vi "Word_doc.vi"(4 "end":i32, 6 "start":i32, 7 "insertion point":u16(ring)=1 items=["begining of document", "end of document", "bookmark", "Custom"], 8 "error in (no error)":errorcluster, 9 "report file path out":path=path "C:/Users/Joseph/Desktop/New folder/5.docx", 10 "Report in 2":path=path "C:/Users/Joseph/Desktop/RRATP000001 ATP_NAMER_60A_BDLC_60A _Vers 10_160816.doc", 11 "Report in 1":path=path "C:/KineticksTester/N30_00000_200817_1048.docx") -> (0 "error out":errorcluster)   [LabVIEW 2017]
uses:
  <vilib>/Utility/NIReport.llb/NI_report.lvclass
  <vilib>/Utility/NIReport.llb/Word/NI_Word.lvclass
  <vilib>/addons/_office/NI_ReportGenerationToolkit.lvlib
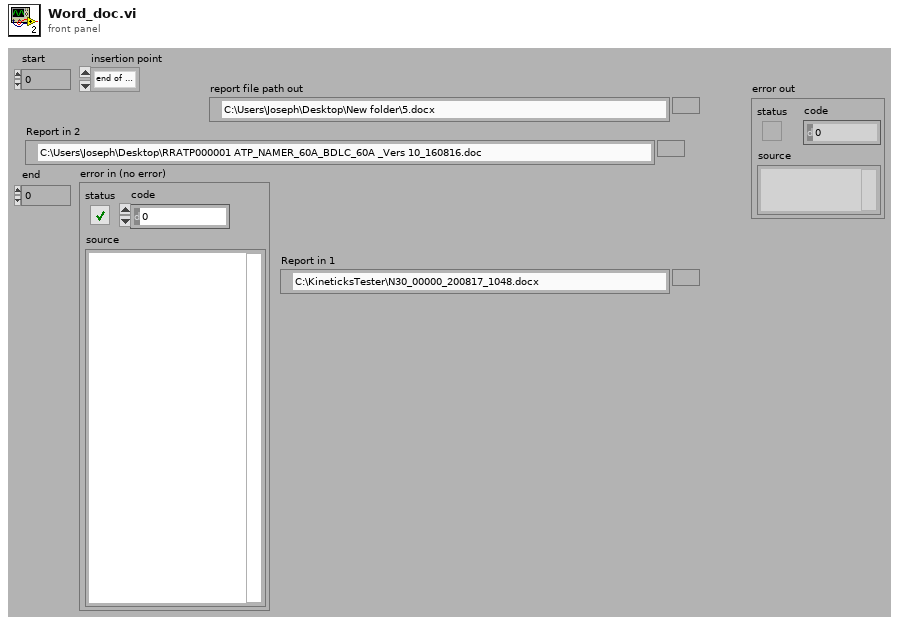
[diagram p1: front panel]
types:
  T1 = enum16{"Standard Report", "HTML", "Word", "Excel"}
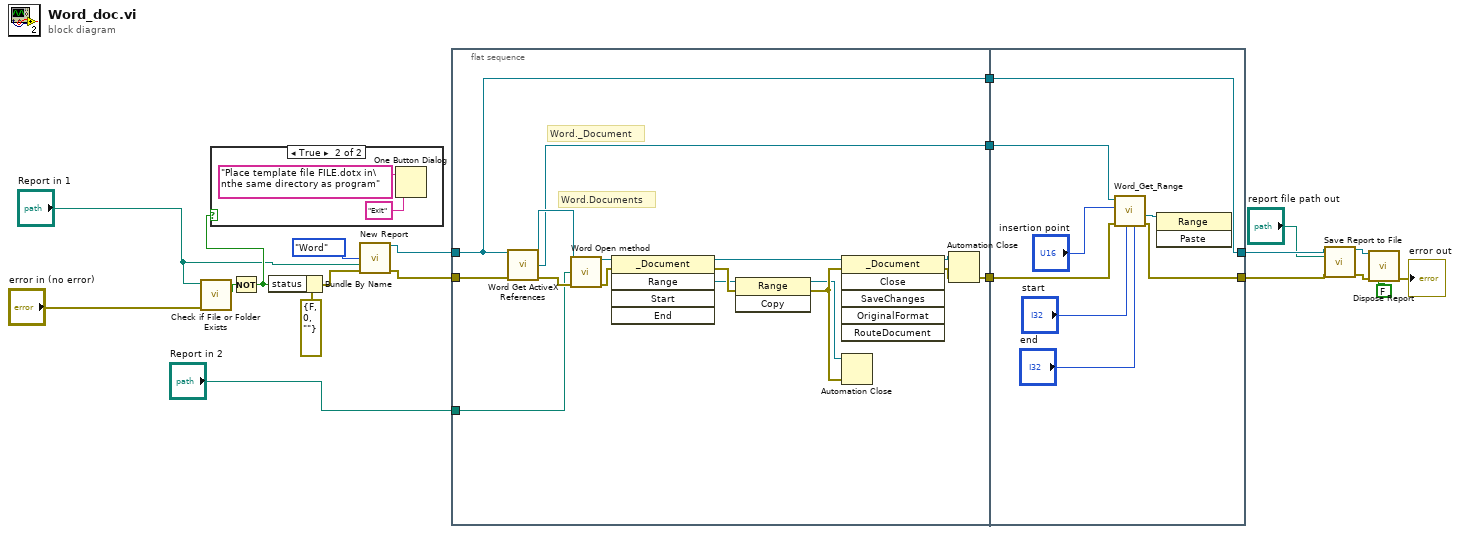
[diagram p0: block diagram]
diagram:
  n1 = call <vilib>:"Check if File or Folder Exists.vi"("error in (no error)"="error in (no error)", "path"="Report in 1") -> ("file or folder exists?"=w17:bool)  [unwired: 7 in, 2 out]
  n2 = Not(x=w17) -> (.not. x?=w13:bool)
  n3 = case shown="True" w13 {
    frame False {
    }
    frame True {
      n4 = One Button Dialog(message="Place template file FILE.dotx in\nthe same directory as program", button name ("OK")="Exit") -> ()  [unwired: 1 out]
    }
  }
  n5 = Bundle By Name(cluster=errorcluster {"status"=FALSE, "code"=0, "source"=""} ("error in (no error)"), "status"=w13) -> (w18:errorcluster)
  n6 = call <vilib>:"New Report.vi"("report type"=T1."Word", "template (empty)"="Report in 1", "error in (no error)"=w18) -> ("report out"=w16:refnum<class "NI_report.lvclass">, "error out"=w15:errorcluster)  [unwired: 11 in]
  n7 = flat-sequence {
    tunnel: w16 -> [w24]
    tunnel: w15 -> [w38]
    tunnel: [w25] -> w12
    tunnel: [w26] -> w11
    tunnel: [w24] -> w10
    tunnel: "Report in 2" -> [w23]
    tunnel: w12 -> [w44]
    tunnel: [w42] -> w7
    tunnel: [w41] -> w6
    tunnel: w11 -> [w43]
    tunnel: w10 -> [w42]
    frame #0 {
      # "Word.Documents"
      # "Word._Document"
      n8 = call <vilib>:"Word Get ActiveX References.vi"("report in"=w24, "error in (no error)"=w38) -> ("Word.Documents"=w29:refnum<k7>, "Word._Document"=w26:refnum<k7>, "error out"=w34:errorcluster)  [unwired: 7 in, 4 out]
      n9 = call <vilib>:"Word Open method.vi"("Word.Documents"=w29, "FileName"=w23, "error in (no error)"=w34) -> ("Open"=w30:refnum<k7>, "error out"=w35:errorcluster)  [unwired: 11 out]
      n10 = invoke on="Range" class="_Document" method="Range"(reference=w30, error in=w35) -> (reference out=w31:refnum<k7>, error out=w33:errorcluster, "Range"=w28:refnum<k7>)  [unwired: 3 in, 2 out]
      n11 = invoke on="Copy" class="Range" method="Copy"(reference=w28, error in=w33) -> (reference out=w27:refnum<k7>, error out=w37:errorcluster)  [unwired: 1 in, 1 out]
      n12 = invoke on="Close" class="_Document" method="Close"(reference=w31, error in=w37) -> (reference out=w32:refnum<k7>, error out=w36:errorcluster)  [unwired: 4 in, 4 out]
      n13 = Automation Close(3:w37, 5:w27) -> ()  [unwired: 1 out]
      n14 = Automation Close(3:w36, 5:w32) -> (0:w25:errorcluster)
    }
    frame #1 {
      n15 = call <vilib>:"Word_Get_Range.vi"("end"="end", "start"="start", "error in"=w44, "insertion point"="insertion point", "document in"=w43) -> ("error out (no error)"=w41:errorcluster, "range"=w45:refnum<k7>)  [unwired: 1 in, 4 out]
      n16 = invoke class="Range" method="Paste"(reference=w45) -> ()  [unwired: 2 in, 3 out]
    }
  }
  n17 = call-dynamic "Save Report to File.vi"("report in"=w7, "report file path"="report file path out", "error in (no error)"=w6) -> ("report out"=w4:refnum<class "NI_report.lvclass">, "error out"=w5:errorcluster)  [unwired: 11 in]
  n18 = call-dynamic "Dispose Report.vi"("report in"=w4, "error in (no error)"=w5, "close report? (T)"=FALSE) -> ("error out"=→"error out":errorcluster)  [unwired: 12 in]
